vi "Write Defect Identify data.vi"(7 "Send any changes now? (F)":bool, 8 "error in (no error)":errorcluster, 10 "Defect Identify data":cluster{"Image":T1, "Measure Report":string}, 11 "Fiber Auto Collimation state data in":refnum<class "Fiber Auto Collimation state data.lvclass">) -> (0 "error out":errorcluster, 3 "Fiber Auto Collimation state data out":refnum<class "Fiber Auto Collimation state data.lvclass">)   [LabVIEW 2018, in "Fiber Auto Collimation state data.lvclass"]
uses:
  Fiber Auto Collimation state data.lvclass
  <vilib>/vision/Image Controls.llb/IMAQ Image.ctl
  Tracked state data.ctl
  Fiber Auto Collimation state data.lvclass/Fiber Auto Collimation state data.ctl
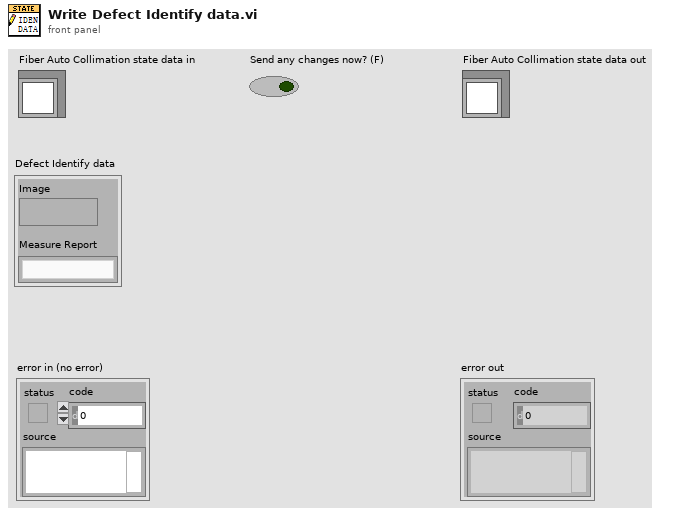
[diagram p1: front panel]
types:
  T1 = typedef "IMAQ Image.ctl" = refnum<image>
  T2 = typedef "Fiber Auto Collimation state data.lvclass/Tracked state data.ctl" = enum16{"No update", "Permission level", "Username", "Test running", "DUT Serial", "Test status", "MOM Lot", "Loaded test recipe", "Model case running", "Station status", "BV data", "Defect Identify data", "Axis Position data", "Fiber Ass PN", "Operator", "RunTime", "VBAI", "Steps Cycle Time"}
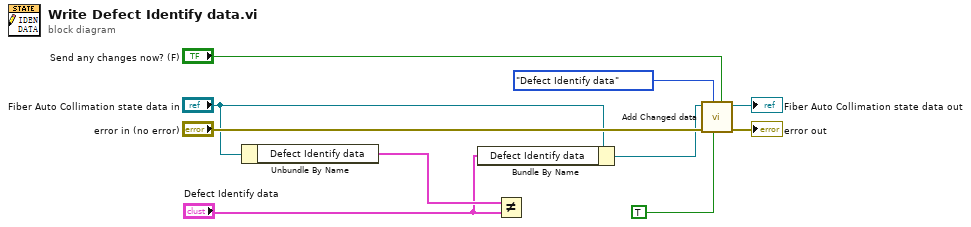
[diagram p0: block diagram]
diagram:
  n1 = Unbundle By Name("Fiber Auto Collimation state data in") -> ("Defect Identify data"=w4:cluster{"Image":T1, "Measure Report":string})
  n2 = Bundle By Name(cluster="Fiber Auto Collimation state data in", "Defect Identify data"="Defect Identify data") -> (w7:refnum<class "Fiber Auto Collimation state data.lvclass">)
  n3 = Not Equal?(x=w4, y="Defect Identify data") -> ()  [unwired: 1 out]
  n4 = call "Add Changed data.vi"("Send any changes now? (F)"="Send any changes now? (F)", "Data changed?"=TRUE, "Data type"=Tracked_state_data."Defect Identify data", "error in (no error)"="error in (no error)", "Fiber Auto Collimation state data in"=w7) -> ("error out"=→"error out":errorcluster, "Fiber Auto Collimation state data out"=→"Fiber Auto Collimation state data out":refnum<class "Fiber Auto Collimation state data.lvclass">)  [unwired: 5 in]
